vi "set_extrapolate_settings.vi"(8 "error in (no error)":errorcluster, 10 "extrapolate distance":i32, 11 "TrajectoryMH100122AODRAPS in":refnum<class "TrajectoryMH100122AODRAPS.lvclass">) -> (0 "error out":errorcluster, 3 "TrajectoryMH100122AODRAPS out":refnum<class "TrajectoryMH100122AODRAPS.lvclass">)   [LabVIEW 2010, in "TrajectoryMH100122AODRAPS.lvclass"]
uses:
  TrajectoryMH100122AODRAPS.lvclass
  TrajectoryMH100122AODRAPS.lvclass/TrajectoryMH100122AODRAPS.ctl
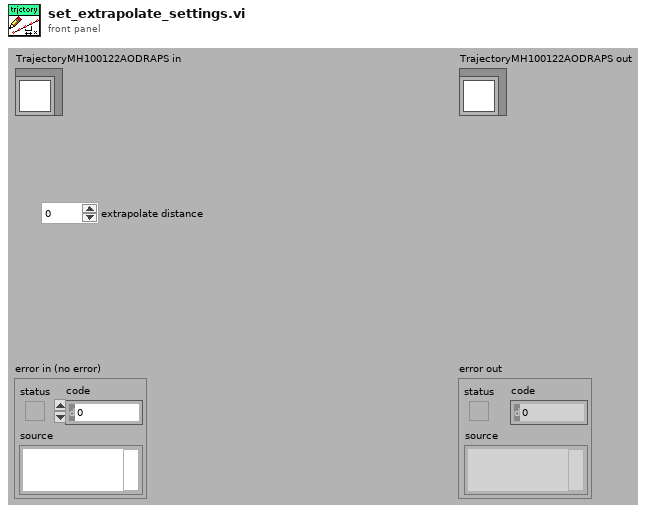
[diagram p1: front panel]
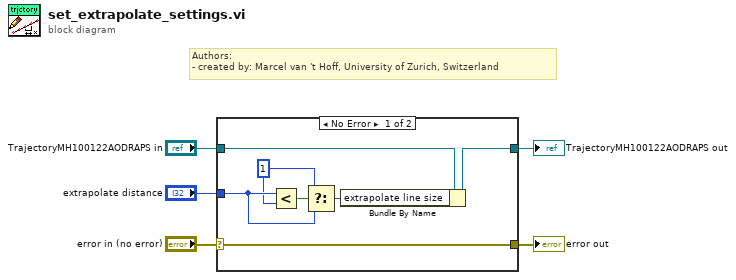
[diagram p0: block diagram]
diagram:
  # "Authors: \n- created by: Marcel van 't Hoff, University of Zurich, Switzerland"
  n1 = case shown="No Error" "error in (no error)" {
    selector: "error in (no error)" -> [w12 w14]
    tunnel: [w12 w14] -> w4
    tunnel: [w10 w13] -> w2
    tunnel: "TrajectoryMH100122AODRAPS in" -> [w11 w13]
    tunnel: "extrapolate distance" -> [w8 _]
    frame No Error {
      w7 = 1 ("t")
      n2 = Less?(x=w8, y=w7) -> (x < y?=w6:bool)
      n3 = Select(t=w7, s=w6, f=w8) -> (s? t:f=w9:i32)
      n4 = Bundle By Name(cluster=w11, "extrapolate line size"=w9) -> (w10:refnum<class "TrajectoryMH100122AODRAPS.lvclass">)
    }
    frame Error {
    }
  }
  "error out" <- w4
  "TrajectoryMH100122AODRAPS out" <- w2
